vi "Probe.vi"(11 "AER Left":refnum<class "AER.lvclass">) -> (2 "Value String":string, 3 "Boolean":bool)   [LabVIEW 2016, in "AER.lvclass"]
uses:
  AER.lvclass
  AER.lvclass/AER.ctl
panel:
  out "Firing rate":cluster{i32, dbl, dbl[]}[](graph)
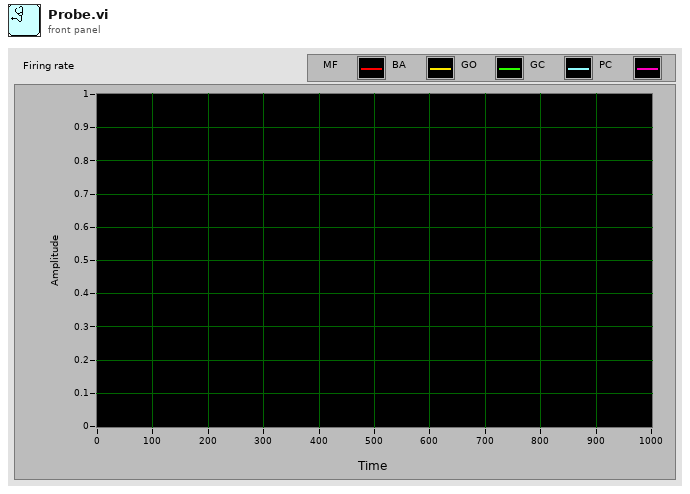
[diagram p1: front panel]
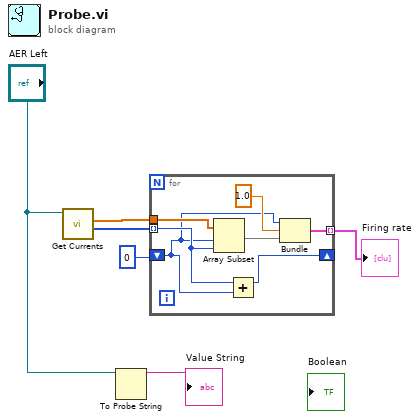
[diagram p0: block diagram]
diagram:
  n1 = call "Get Currents.vi"("AER in"="AER Left") -> ("No N"=w4:i32[], "Currents"=w3:dbl[])  [unwired: 8 in, 1 out]
  n2 = To Probe String(7:"AER Left") -> (3:→"Value String":string)  [unwired: 2 in, 1 out]
  n3 = for {
    tunnel: w4 -> [w12] mode=indexing
    tunnel: w3 -> [w13]
    shift-right: [w8] -> _
    shift-left: 0 -> [w7]
    tunnel: [w9] -> w1 mode=indexing
    n4 = Array Subset(array=w13, index=w7, length=w12) -> (w11:dbl[])
    n5 = Add(x=w12, y=w7) -> (x+y=w8:i32)
    n6 = Bundle(w7, 1.0, w11) -> (w9:cluster{i32, dbl, dbl[]})  [unwired: 1 in]
  }
  "Firing rate" <- w1
